vi "Instrument.TestLauncher.vi"() -> ()   [LabVIEW 2016, in "Instrument.lvclass"]
uses:
  Instrument.lvclass
  <vilib>/JKI/JKI SMO/SMO/Typedefs/SMOState --Enum.ctl
  Typedefs/PrivateEvents--Instrument.SetPort.ctl
  Typedefs/PrivateEvents--Instrument.SetCommands.ctl
  Typedefs/PrivateEvents--Instrument.SetAllowedRemote.ctl
  C:/Program Files (x86)/National Instruments/LabVIEW 2016/vi.lib/JKI/JKI SMO/SMO/SMO.lvclass
  <vilib>/JKI/JKI SMO/SMO/SMO.lvclass
panel:
  in  "SetAllowedRemote":T1
  in  "SetCommands":T2=["Command1", "Command2"]
  in  "SetPort":T3=6341
  out "SMO State":T4=enum."Stopped"
  out "error out":errorcluster
  in  "Stop":bool
  # "Instrument SMO Test Launcher"
  # "For instructions on how to use the JKI State Machine Objects, examples and video tutorials, visit:\nhttp://jki.net/state-machine-objects/\n\nJKI State Machine Objects™\nhttp://jki.net/state-machine-objects/\nCopyright (C) 2005-2015, JKI <info@jki.net>\nALL RIGHTS RESERVED"
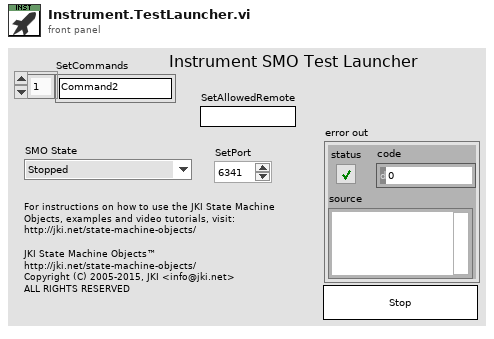
[diagram p1: front panel]
types:
  T1 = typedef "Instrument.lvclass/PrivateEvents--Instrument.SetAllowedRemote.ctl" = string
  T2 = typedef "Instrument.lvclass/PrivateEvents--Instrument.SetCommands.ctl" = string[]
  T3 = typedef "Instrument.lvclass/PrivateEvents--Instrument.SetPort.ctl" = i32
  T4 = typedef "SMO.lvclass/SMOState --Enum.ctl" = enum16{"unknown", "Created", "Started", "Stopped"}
  T5 = typedef "SMO.lvclass/Public Events.ctl" = cluster{"Error":refnum<user-event>, "State":refnum<user-event>, "Reserve State":refnum<user-event>}
  T6 = cluster{"Event Registration Refnum":refnum<event-registration>}
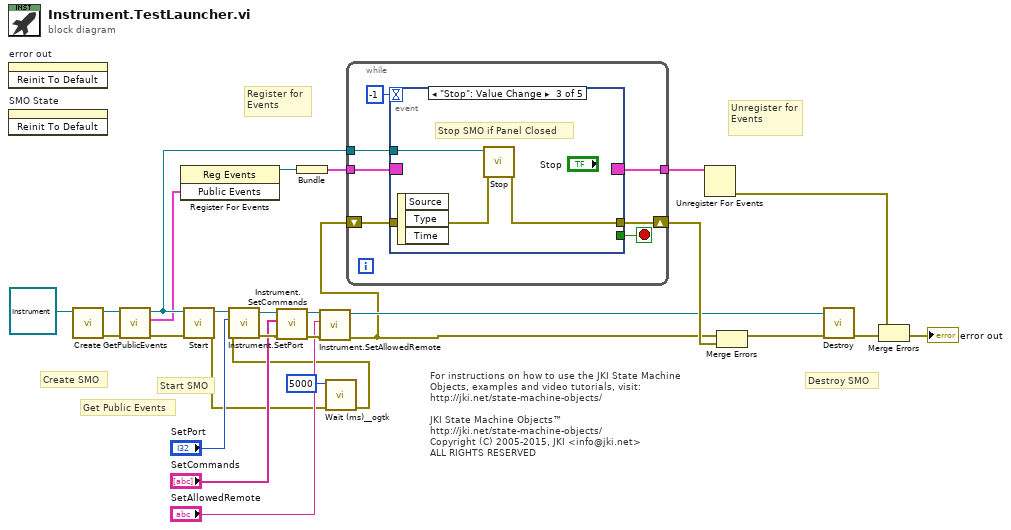
[diagram p0: block diagram]
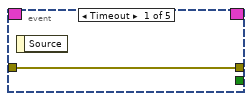
[diagram p2: hidden frame]
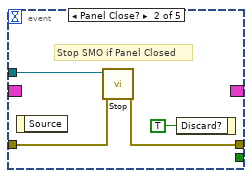
[diagram p3: hidden frame]
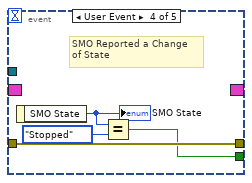
[diagram p4: hidden frame]
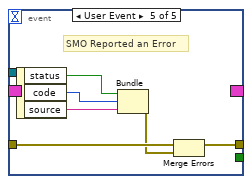
[diagram p5: hidden frame]
diagram:
  # "For instructions on how to use the JKI State Machine Objects, examples and video tutorials, visit:\nhttp://jki.net/state-machine-objects/\n\nJKI State Machine Objects™\nhttp://jki.net/state-machine-objects/\nCopyright (C) 2005-2015, JKI <info@jki.net>\nALL RIGHTS RESERVED"
  # "Get Public Events"
  # "Start SMO"
  # "Destroy SMO"
  # "Create SMO"
  # "Unregister for Events"
  # "Register for Events"
  n1 = invoke on="error out" class="Clust (strict)" method="Reinit To Default"() -> ()  [unwired: 3 in, 3 out]
  n2 = invoke on="SMO State" class="Enum (strict)" method="Reinit To Default"() -> ()  [unwired: 3 in, 3 out]
  n3 = call <vilib>:"Create.vi"("SMO"=refnum<class "Instrument.lvclass"> refnum ("SMO.Template.lvclass")) -> ("error out"=w18:errorcluster, "SMO out"=w19:refnum<class "Instrument.lvclass">)  [unwired: 8 in, 1 out]
  n4 = call <vilib>:"GetPublicEvents.vi"("error in (no error)"=w18, "SMO"=w19) -> ("error out"=w17:errorcluster, "Public Events"=w15:T5, "SMO out"=w16:refnum<class "Instrument.lvclass">)  [unwired: 7 in]
  n5 = register-events(w15) -> (reference out=w14:refnum<event-registration>)  [unwired: 2 in, 1 out]
  n6 = call <vilib>:"Start.vi"("error in (no error)"=w17, "SMO"=w16) -> ("error out"=w3:errorcluster, "SMO out"=w13:refnum<class "Instrument.lvclass">)  [unwired: 8 in]
  n7 = Bundle("Event Registration Refnum"=w14) -> (w26:T6)  [unwired: 1 in]
  n8 = call <userlib>:"Wait (ms)__ogtk.vi"("error in (no error)"=w3, "milliseconds to wait"=u32 5000) -> ("error out"=w2:errorcluster)  [unwired: 8 in, 1 out]
  n9 = call "Instrument.SetPort.vi"("error in (no error)"=w2, "Write Port"="SetPort", "Instrument"=w13) -> ("error out"=w12:errorcluster, "Instrument out"=w11:refnum<class "Instrument.lvclass">)  [unwired: 7 in]
  n10 = call "Instrument.SetCommands.vi"("error in (no error)"=w12, "Write Commands"="SetCommands", "Instrument"=w11) -> ("error out"=w10:errorcluster, "Instrument out"=w9:refnum<class "Instrument.lvclass">)  [unwired: 7 in]
  n11 = call "Instrument.SetAllowedRemote.vi"("error in (no error)"=w10, "Write Allowed Remote"="SetAllowedRemote", "Instrument"=w9) -> ("error out"=w6:errorcluster, "Instrument out"=w7:refnum<class "Instrument.lvclass">)  [unwired: 7 in]
  n12 = while {
    shift-right: [w33] -> w25
    shift-left: w6 -> [w32]
    tunnel: w26 -> [w31]
    tunnel: [w30] -> w27
    tunnel: w16 -> [w29]
    stop <- w34 stop-if-true
    n13 = event shown="[2] \"Stop\": Value Change" {
      selector: w31 -> [_ _ _ _ _]
      dyn-events: [_ _ _ _ _] -> w30
      timeout: -1 -> [_ _ _ _ _]
      tunnel: [_ _ _ w43 _] -> w34
      tunnel: w29 -> [_ w39 w42 _ _]
      tunnel: [w35 w38 w41 w46 w50] -> w33
      tunnel: w32 -> [w35 w37 w40 w46 w48]
      event Timeout {
        n14 = event-data() -> ()  [unwired: 1 in, 1 out]
      }
      event Panel Close? {
        # "Stop SMO if Panel Closed"
        n15 = event-data() -> ()  [unwired: 1 in, 1 out]
        n16 = call <vilib>:"Stop.vi"("error in (no error)"=w37, "SMO"=w39) -> ("error out"=w38:errorcluster)  [unwired: 8 in, 1 out]
        n17 = event-data("Discard?"=TRUE ("OK")) -> ()  [unwired: 1 in, 1 out]
      }
      event "Stop": Value Change {
        # "Stop SMO if Panel Closed"
        n18 = event-data() -> ()  [unwired: 1 in, 3 out]
        n19 = call <vilib>:"Stop.vi"("error in (no error)"=w40, "SMO"=w42) -> ("error out"=w41:errorcluster)  [unwired: 8 in, 1 out]
      }
      event User Event {
        # "SMO Reported a Change\nof State"
        n20 = event-data() -> ("SMO State"=w45:T4)  [unwired: 1 in]
        "SMO State" <- w45
        n21 = Equal?(x=w45, y=SMOState_--Enum."Stopped") -> (x = y?=w43:bool)
      }
      event User Event {
        # "SMO Reported an Error"
        n22 = event-data() -> ("status"=w49:bool, "code"=w52:i32, "source"=w51:string)  [unwired: 1 in]
        n23 = Bundle("status"=w49, "code"=w52, "source"=w51) -> (w47:errorcluster)  [unwired: 1 in]
        n24 = Merge Errors(w48, w47) -> (w50:errorcluster)
      }
    }
  }
  n25 = Unregister For Events(event registration refnum=w27) -> (error out=w24:errorcluster)  [unwired: 1 in]
  n26 = Merge Errors(w6, w25) -> (w20:errorcluster)
  n27 = call <vilib>:"Destroy.vi"("error in (no error)"=w20, "SMO"=w7) -> ("error out"=w22:errorcluster)  [unwired: 9 in]
  n28 = Merge Errors(w24, w22) -> (→"error out":errorcluster)
